vi "Get Nest Aliases.vi"(7 "Actor":refnum<class "LVCAM.lvclass">) -> (0 "error out":errorcluster, 2 "Nest Aliases":string[](array[string]))   [LabVIEW 2021, in "LVCAM.lvlib" / "Actor.lvclass"]
uses:
  Actor.lvclass
  LVCAM/LVCAM.lvclass
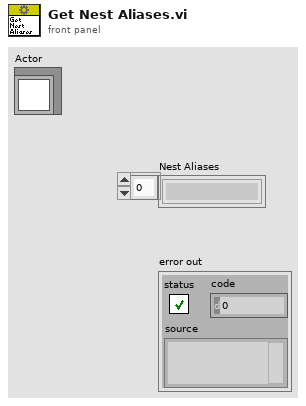
[diagram p1: front panel]
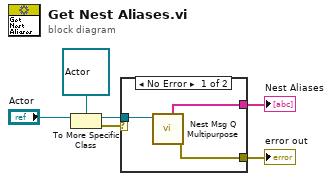
[diagram p0: block diagram]
diagram:
  n1 = To More Specific Class(target class=refnum<class "Actor.lvclass"> refnum ("LVCAM.lvlib:Self Actor.lvclass"), reference="Actor") -> (specific class reference=w4:refnum<class "Actor.lvclass">, error out=w2:errorcluster)  [unwired: 1 in]
  n2 = case shown="No Error" w2 {
    selector: w2 -> [_ w10]
    tunnel: [w9 w10] -> w1
    tunnel: [w7 _] -> w6
    tunnel: w4 -> [w8 _]
    frame No Error {
      n3 = call "Nest Msg Q Multipurpose.vi"("Actor in"=w8) -> ("error out"=w9:errorcluster, "Nest Aliases"=w7:string[])  [unwired: 6 in, 3 out]
    }
    frame Error {
      # "#TypeCastError"
    }
  }
  "error out" <- w1
  "Nest Aliases" <- w6
